vi "Acquire Waveform.vi"(8 "error in (no error)":errorcluster, 11 "DAQ AI in":refnum<class "DAQ AI.lvclass">) -> (0 "error out":errorcluster, 3 "DAQ AI out":refnum<class "DAQ AI.lvclass">)   [LabVIEW 2020, in "DAQ AI.lvlib" / "DAQ AI.lvclass"]
uses:
  DAQ AI.lvclass
  DAQ AI.lvclass/DAQ AI.ctl
  <vilib>/DAQmx/read.llb/DAQmx Read (Analog 1D Wfm NChan NSamp).vi
  <vilib>/measure/NI_MABase.lvlib
  <vilib>/numeric/Random Number (Range) DBL.vi
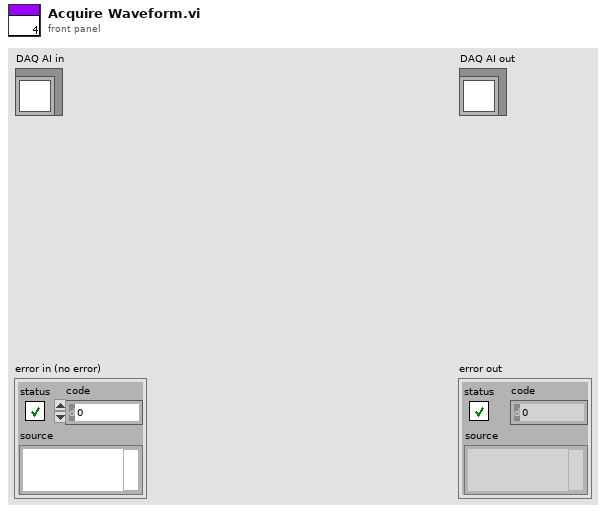
[diagram p1: front panel]
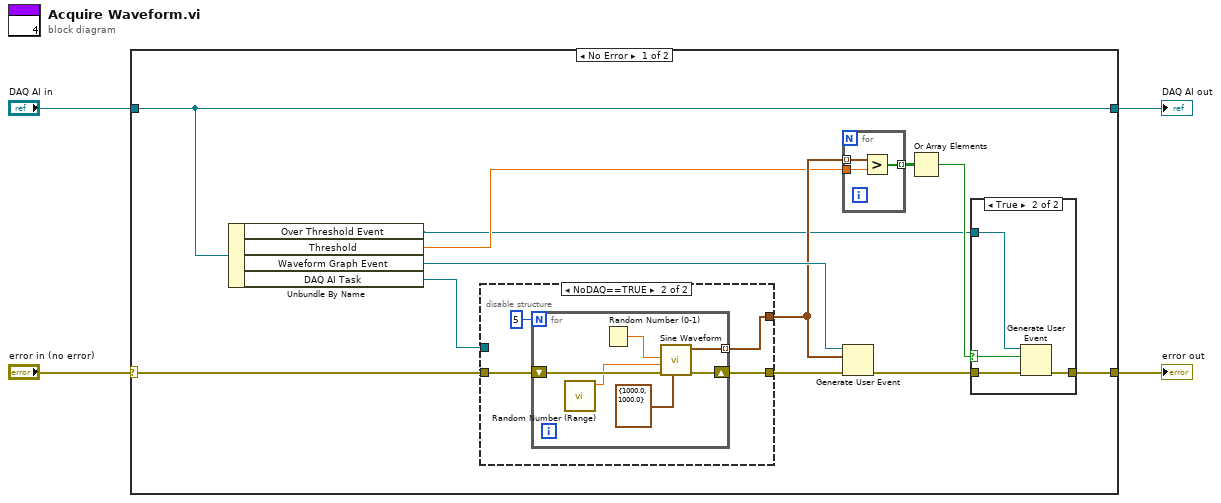
[diagram p0: block diagram]
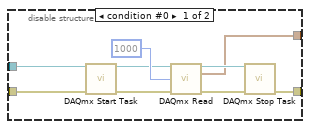
[diagram p2: hidden frame]
diagram:
  n1 = case shown="No Error" "error in (no error)" {
    selector: "error in (no error)" -> [w13 w45]
    tunnel: [w7 w45] -> w3
    tunnel: [w16 w44] -> w1
    tunnel: "DAQ AI in" -> [w16 w44]
    frame No Error {
      n2 = Unbundle By Name(w16) -> ("Over Threshold Event"=w5:refnum<user-event>, "Threshold"=w10:dbl, "Waveform Graph Event"=w15:refnum<user-event>, "DAQ AI Task"=w14:refnum<k21>)
      n3 = disable-structure shown="NoDAQ==TRUE" {
        disable-tunnel: w14 -> [w24 _]
        disable-tunnel: w13 -> [w22 w29]
        disable-tunnel: [w18 w27] -> w12
        disable-tunnel: [w17 w26] -> w11
        frame condition #0 {
          n4 = call <vilib>:"DAQmx Start Task.vi"("task/channels in"=w24, "error in"=w22) -> ("task out"=w23:refnum<k21>, "error out"=w21:errorcluster)  [unwired: 12 in]
          n5 = call-poly <vilib>:"DAQmx Read.vi"("task/channels in"=w23, "number of samples per channel"=1000, "error in"=w21) -> ("task out"=w20:refnum<k21>, "data"=w17:waveform(dbl)[], "error out"=w19:errorcluster)  [unwired: 10 in]
          n6 = call <vilib>:"DAQmx Stop Task.vi"("task/channels in"=w20, "error in"=w19) -> ("error out"=w18:errorcluster)  [unwired: 12 in, 1 out]
        }
        frame condition #1 (active) {
          n7 = for {
            N: 5 -> [_]
            shift-right: [w33] -> w27
            shift-left: w29 -> [w34]
            tunnel: [w32] -> w26 mode=indexing
            n8 = call-poly <vilib>:"Random Number (Range).vi"() -> ("number"=w30:dbl)  [unwired: 11 in]
            n9 = Random Number (0-1)() -> (number: 0 to 1=w31:dbl)
            n10 = call <vilib>:"Sine Waveform.vi"("sampling info"=cluster{"Fs":dbl, "#s":dbl} {"Fs"=1000.0, "#s"=1000.0}, "error in (no error)"=w34, "phase"=w30, "amplitude"=w31) -> ("error out"=w33:errorcluster, "signal out"=w32:waveform(dbl))  [unwired: 6 in]
          }
        }
      }
      n11 = for {
        tunnel: w11 -> [w43] mode=indexing
        tunnel: w10 -> [w42]
        tunnel: [w41] -> w9 mode=indexing
        n12 = Greater?(x=w43, y=w42) -> (0:w41:bool[])
      }
      n13 = Generate User Event(user event=w15, event data cluster=w11, error in=w12) -> (error out=w8:errorcluster)  [unwired: 1 in, 1 out]
      n14 = Or Array Elements(Boolean array=w9) -> (logical OR=w6:bool)
      n15 = case shown="True" w6 {
        selector: w6 -> [_ w38]
        tunnel: w8 -> [w36 w40]
        tunnel: [w36 w39] -> w7
        tunnel: w5 -> [_ w37]
        frame False {
        }
        frame True {
          n16 = Generate User Event(user event=w37, event data cluster=w38, error in=w40) -> (error out=w39:errorcluster)  [unwired: 1 in, 1 out]
        }
      }
    }
    frame Error {
    }
  }
  "error out" <- w3
  "DAQ AI out" <- w1
